vi "Select Sheet by Name.vi"(7 "Sheet (Sheet1)":string="Sheet1", 8 "error in (no error)":errorcluster, 11 "Excel XML in":refnum<class "Excel XML.lvclass">) -> (0 "error out":errorcluster, 3 "Excel XML out":refnum<class "Excel XML.lvclass">)   [LabVIEW 2013, in "Excel XML.lvclass"]
uses:
  Excel XML.lvclass
  Spreadsheet.lvclass
  Excel XML.lvclass/Excel XML.ctl
  C:/PhaeronGit/LVNPOI/Resources/NPOI 2.1.1 dotnet4/NPOI.OOXML.dll
  Resources/NPOI 2.1.1 dotnet4/NPOI.OOXML.dll
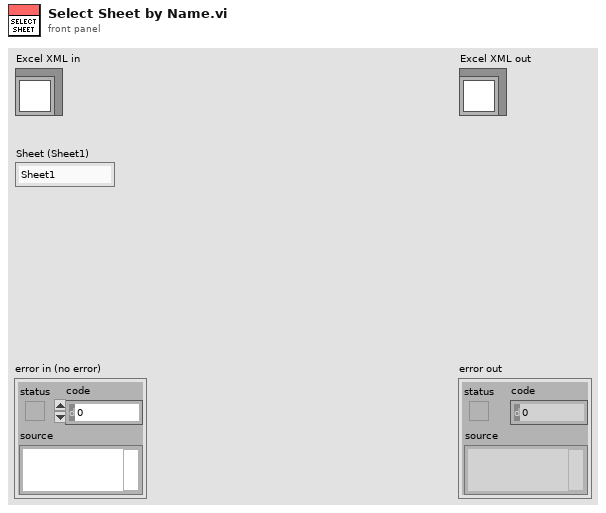
[diagram p1: front panel]
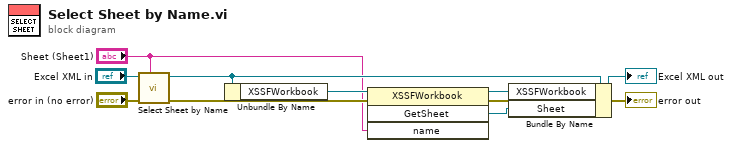
[diagram p0: block diagram]
diagram:
  n1 = call-parent "Select Sheet by Name.vi"("Sheet (Sheet1)"="Sheet (Sheet1)", "error in (no error)"="error in (no error)", "Spreadsheet in"="Excel XML in") -> ("error out"=w5:errorcluster, "Spreadsheet out"=w3:refnum<class "Excel XML.lvclass">)  [unwired: 7 in]
  n2 = Unbundle By Name(w3) -> ("XSSFWorkbook"=w6:refnum<k24>)
  n3 = invoke class="XSSFWorkbook" method="GetSheet"(reference=w6, error in=w5, "name"="Sheet (Sheet1)") -> (reference out=w7:refnum<k24>, error out=→"error out":errorcluster, "GetSheet"=w8:refnum<k24>)  [unwired: 1 in, 1 out]
  n4 = Bundle By Name(cluster=w3, "XSSFWorkbook"=w7, "Sheet"=w8) -> (→"Excel XML out":refnum<class "Excel XML.lvclass">)
